vi "find_speedup.vi"(7 "Parameters":T2={"Stimulus"={"Type"=enum."Off", "Phase"=0.0, "Amplitude"=[], "Injection point"=enum."Total pose", "Closed loop"=FALSE, "Offset"=[], "Tip -> world"=FALSE, "Frequency"=0.0, "Length"=0.0}, "Goal Filter A"={"Speedup max"=0.0, "Speedup thresh"=0.0, "Speedup nonlin"=0.0, "Filters"=[]}, "Mode controls"={"Hold"=FALSE, "Cancellation"=FALSE, "Goal filter"=FALSE, "Trigger"=FALSE}, "Manipulator type"=enum."Current piezo", "Manipulator calibration"={"Tool offsets"=[[0.0, 0.0, 36200.0]], "Handle light calibration"=[], "Base pivots"=[], "Output pivots"=[], "Length center"=0.0, "Workspace height"=[], "Workspace diameter"=[0.0, 0.0, 36200.0], "Stack travel"=400.0, "Saturation pos"=375.0, "Inverse filters"=[], "Strut length"=0.0}, "Network"={"Remote Host"="", "Send Status"=FALSE, "Send Port"=0, "Recv Commands"=FALSE, "Recv Port"=0}, "Goal Filter B"={"Speedup max"=0.0, "Speedup thresh"=0.0, "Speedup nonlin"=0.0, "Filters"=[]}, "Cancellation"={"KP"={"XY"=0.0, "Rxy"=0.0, "Z"=0.0, "Rz"=0.0}, "KI"=0.0, "KD"={"XY"=0.0, "Rxy"=0.0, "Z"=0.0, "Rz"=0.0}, "Max vel"=20.0, "Max acc"=0.001, "Int error limit"=3.0, "RCM gain"=0.0, "Bypass"=FALSE, "Degraded gain"=0.0}, "Transition time"=0.0, "Estimation"={"Link"={"Measure noise"=[], "Process noise"=[], "Alt process noise"=[], "Alt turnoff cycles"=20, "Innovation limit"=[], "Residue threshold"=0.0, "Enable"=FALSE}, "Handle"={"Measure noise"=[], "Process noise"=[], "State limits"=[], "Innovation limit"=[], "Prediction Lookahead"=0.0, "Enable"=FALSE}}} {"Transition time" format="%_3f"; "Cancellation"."Degraded gain" min=0 max=1 step=0.1 format="%#_3p"; "Cancellation"."RCM gain" min=0 max=1 step=0.1 format="%#_3p"; "Cancellation"."KD"."Rz" min=-1 max=1 step=0.01 format="%#_3p"; "Cancellation"."KD"."Rxy" min=-1 max=1 step=0.01 format="%#_3p"; "Cancellation"."KD"."Z" min=-1 max=1 step=0.01 format="%#_3p"; "Cancellation"."KD"."XY" min=-1 max=1 step=0.01 format="%#_3p"; "Cancellation"."KI" min=0 max=1 step=0.01 format="%#_3p"; "Cancellation"."KP"."Rz" min=-1 max=1 step=0.01 format="%#_3p"; "Cancellation"."KP"."Rxy" min=-1 max=1 step=0.01 format="%#_3p"; "Cancellation"."KP"."Z" min=-1 max=1 step=0.01 format="%#_3p"; "Cancellation"."KP"."XY" min=-1 max=1 step=0.01 format="%#_3p"; "Cancellation"."Max acc" format="%#_3p"; "Goal Filter B"."Filters"."V limit range" format="%_3p"; "Goal Filter B"."Filters"."V limit" format="%_3p"; "Goal Filter B"."Filters"."Upper Q" format="%_3f"; "Goal Filter B"."Filters"."Upper Fc" format="%_3p"; "Goal Filter B"."Filters"."Lower Q" format="%_3f"; "Goal Filter B"."Filters"."Scale factor" format="%_3f"; "Goal Filter B"."Filters"."Lower Fc" format="%_3p"; "Goal Filter B"."Speedup nonlin" format="%_3p"; "Goal Filter B"."Speedup thresh" format="%_3p"; "Goal Filter B"."Speedup max" format="%_3p"; "Manipulator calibration"."Strut length" format="%#_4p"; "Manipulator calibration"."Saturation pos" format="%#.1f"; "Manipulator calibration"."Stack travel" format="%#.1f"; "Manipulator calibration"."Length center" format="%#_4p"; "Manipulator calibration"."Output pivots" format="%#_6f"; "Manipulator calibration"."Base pivots" format="%#_6f"; "Manipulator calibration"."Handle light calibration" format="%#.1f"; "Goal Filter A"."Filters"."V limit range" format="%_3p"; "Goal Filter A"."Filters"."V limit" format="%_3p"; "Goal Filter A"."Filters"."Upper Q" format="%_3f"; "Goal Filter A"."Filters"."Upper Fc" format="%_3p"; "Goal Filter A"."Filters"."Lower Q" format="%_3f"; "Goal Filter A"."Filters"."Scale factor" format="%_3f"; "Goal Filter A"."Filters"."Lower Fc" format="%_3p"; "Goal Filter A"."Speedup nonlin" format="%_3p"; "Goal Filter A"."Speedup thresh" format="%_3p"; "Goal Filter A"."Speedup max" format="%_3p"; "Stimulus"."Length" min=0.0 max=100.0 step=100.0 format="%#_4p"; "Stimulus"."Frequency" min=0.0 step=100.0 format="%#_4g"; "Stimulus"."Offset" format="%#_3p"; "Stimulus"."Amplitude" format="%#_3p"; "Stimulus"."Phase" min=-180.0 max=360.0 step=100.0 format="%#.2f"}, 9 "Goal Filter":T1={"Speedup max"=0.08, "Speedup thresh"=0.606, "Speedup nonlin"=3.0, "Filters"=[]} {"Filters"."V limit range" format="%_3p"; "Filters"."V limit" format="%_3p"; "Filters"."Upper Q" format="%_3f"; "Filters"."Upper Fc" format="%_3p"; "Filters"."Lower Q" format="%_3f"; "Filters"."Scale factor" format="%_3f"; "Filters"."Lower Fc" format="%_3p"; "Speedup nonlin" format="%_3p"; "Speedup thresh" format="%_3p"; "Speedup max" format="%_3p"}, 10 "Stack positions":sgl[](array[numeric])) -> (2 "Speedup":sgl)   [LabVIEW 2014]
uses:
  testing/Micron params.ctl
  testing/stimulus.ctl
  testing/injection_point.ctl
  goal_loop_parms.ctl
  testing/mode_conrols.ctl
  testing/manipulator_cal.ctl
  asap/labview/testing/probe_calibration.ctl
  host/network_params.ctl
  cancellation/sq_control_params.ctl
  cancellation/decoupled_gain.ctl
  cancellation/estimation_controls.ctl
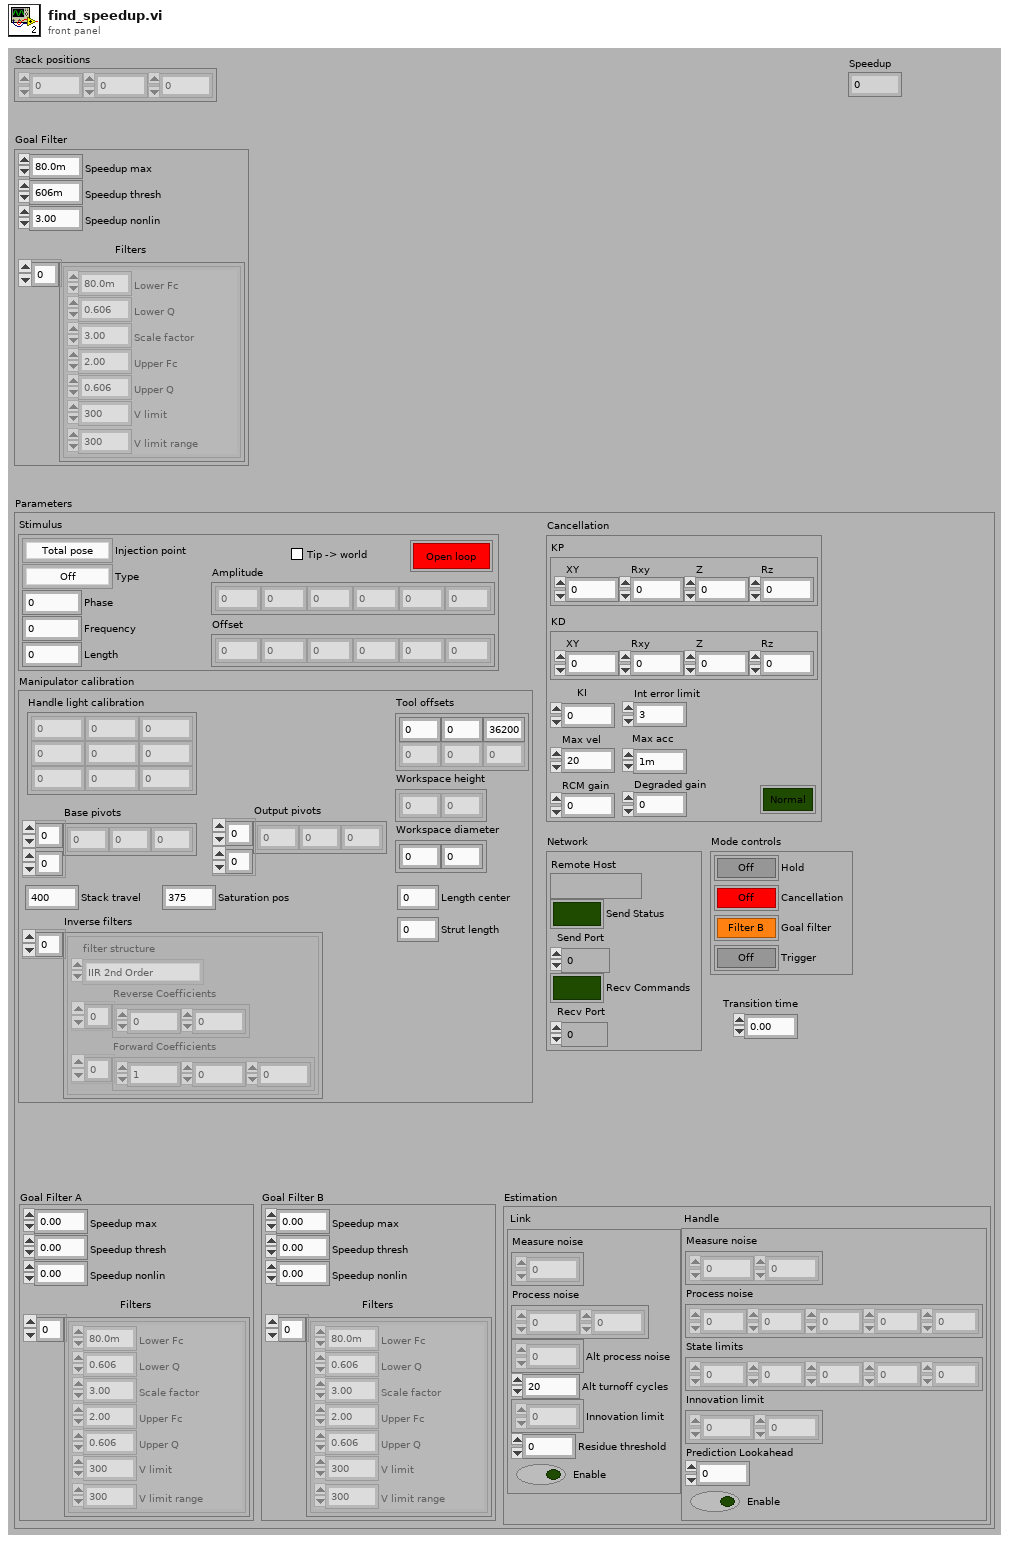
[diagram p1: front panel]
types:
  T1 = typedef "goal_loop_parms.ctl" = cluster{"Speedup max":sgl, "Speedup thresh":sgl, "Speedup nonlin":sgl, "Filters":cluster{"Lower Fc":sgl, "Lower Q":sgl, "Scale factor":sgl, "Upper Fc":sgl, "Upper Q":sgl, "V limit":sgl, "V limit range":sgl}[]}
  T2 = typedef "Micron params.ctl" = cluster{"Stimulus":T3, "Goal Filter A":T1, "Mode controls":T5, "Manipulator type":enum16{"Current piezo", "Voltage piezo"}, "Manipulator calibration":T6, "Network":T8, "Goal Filter B":T1, "Cancellation":T9, "Transition time":sgl, "Estimation":T11}
  T3 = typedef "stimulus.ctl" = cluster{"Type":enum16{"Off", "Step", "Sine", "Triangle", "Arbitrary"}, "Phase":dbl, "Amplitude":sgl[], "Injection point":T4, "Closed loop":bool, "Offset":sgl[], "Tip -> world":bool, "Frequency":dbl, "Length":dbl}
  T4 = typedef "injection_point.ctl" = enum16{"Total pose", "V limiter", "Goal ", "Link position", "KF link position", "Inverse kin", "Link goal", "Link error", "Controller", "Output", "Drive", "Light"}
  T5 = typedef "mode_conrols.ctl" = cluster{"Hold":bool, "Cancellation":bool, "Goal filter":bool, "Trigger":bool}
  T6 = typedef "manipulator_cal.ctl" = cluster{"Tool offsets":sgl[][], "Handle light calibration":T7, "Base pivots":sgl[][], "Output pivots":sgl[][], "Length center":sgl, "Workspace height":sgl[], "Workspace diameter":sgl[], "Stack travel":sgl, "Saturation pos":sgl, "Inverse filters":cluster{"filter structure":enum32{"IIR 2nd Order", "IIR 4th Order"}, "Reverse Coefficients":dbl[], "Forward Coefficients":dbl[]}[], "Strut length":sgl}
  T7 = typedef "probe_calibration.ctl" = sgl[][]
  T8 = typedef "network_params.ctl" = cluster{"Remote Host":string, "Send Status":bool, "Send Port":u16, "Recv Commands":bool, "Recv Port":u16}
  T9 = typedef "sq_control_params.ctl" = cluster{"KP":T10, "KI":sgl, "KD":T10, "Max vel":sgl, "Max acc":sgl, "Int error limit":sgl, "RCM gain":sgl, "Bypass":bool, "Degraded gain":sgl}
  T10 = typedef "decoupled_gain.ctl" = cluster{"XY":sgl, "Rxy":sgl, "Z":sgl, "Rz":sgl}
  T11 = typedef "estimation_controls.ctl" = cluster{"Link":cluster{"Measure noise":dbl[], "Process noise":dbl[], "Alt process noise":dbl[], "Alt turnoff cycles":i32, "Innovation limit":dbl[], "Residue threshold":dbl, "Enable":bool}, "Handle":cluster{"Measure noise":dbl[], "Process noise":dbl[], "State limits":dbl[], "Innovation limit":dbl[], "Prediction Lookahead":sgl, "Enable":bool}}
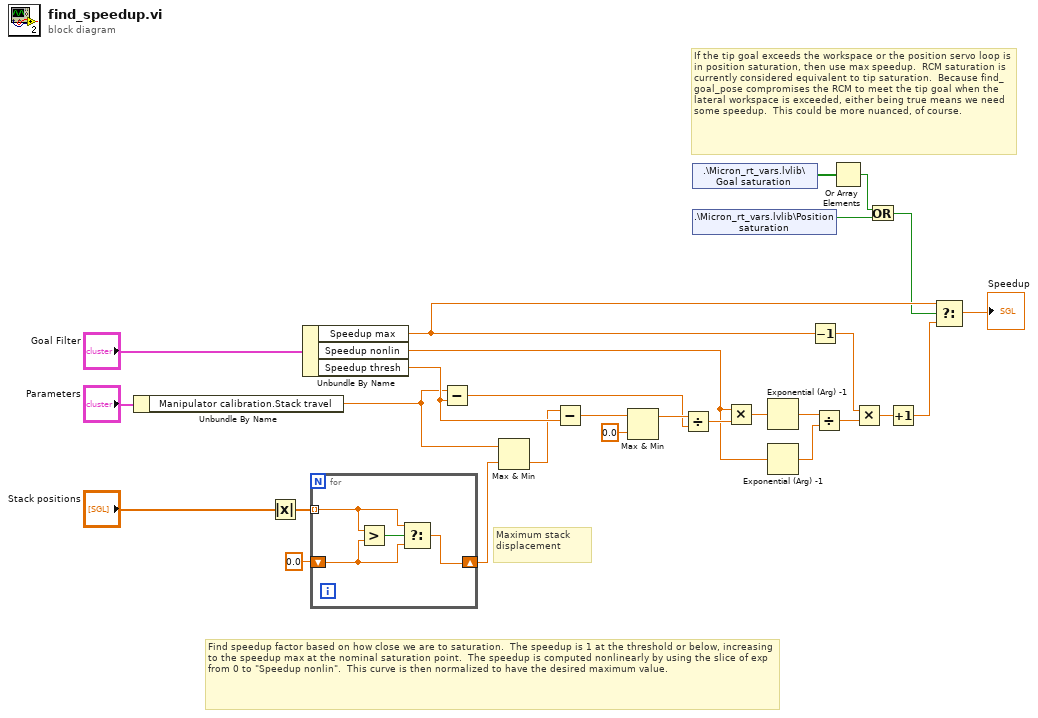
[diagram p0: block diagram]
diagram:
  # "If the tip goal exceeds the workspace or the position servo loop is in position saturation, then use max speedup.  RCM saturation is currently considered equivalent to tip saturation.  Because find_goal_pose compromises the RCM to meet the tip goal when the lateral workspace is exceeded, either being true means we need some speedup.  This could be more nuanced, of course."
  # "Find speedup factor based on how close we are to saturation.  The speedup is 1 at the threshold or below, increasing to the speedup max at the nominal saturation point.  The speedup is computed nonlinearly by using the slice of exp from 0 to \"Speedup nonlin\".  This curve is then normalized to have the desired maximum value."
  # "Maximum stack displacement"
  n1 = Unbundle By Name("Parameters") -> ("Manipulator calibration.Stack travel"=w5:sgl)
  n2 = Absolute Value(x="Stack positions") -> (abs(x)=w27:sgl[])
  n3 = Unbundle By Name("Goal Filter") -> ("Speedup max"=w10:sgl, "Speedup nonlin"=w18:sgl, "Speedup thresh"=w23:sgl)
  n4 = for {
    tunnel: w27 -> [w31] mode=indexing
    shift-right: [w29] -> w9
    shift-left: sgl 0.0 ("Goal Filter.Speedup thresh") -> [w30]
    n5 = Greater?(x=w31, y=w30) -> (0:w32:bool)
    n6 = Select(t=w31, s=w32, f=w30) -> (s? t:f=w29:sgl)
  }
  n7 = Subtract(x=w5, y=w23) -> (x-y=w14:sgl)
  n8 = Max & Min(x=w5, y=w9) -> (min(x,y)=w8:sgl)  [unwired: 1 out]
  n9 = Subtract(x=w8, y=w23) -> (x-y=w22:sgl)
  n10 = Max & Min(x=w22, y=sgl 0.0) -> (max(x,y)=w21:sgl)  [unwired: 1 out]
  n11 = Divide(x=w21, y=w14) -> (x/y=w20:sgl)
  n12 = shared-variable ".\\Micron_rt_vars.lvlib\\Goal saturation"() -> (w2:bool[])  [unwired: 2 out]
  n13 = shared-variable ".\\Micron_rt_vars.lvlib\\Position saturation"() -> (w4:bool)  [unwired: 2 out]
  n14 = Multiply(x=w18, y=w20) -> (x*y=w19:sgl)
  n15 = Exponential (Arg) -1(1:w19) -> (0:w17:sgl)
  n16 = Exponential (Arg) -1(1:w18) -> (0:w16:sgl)
  n17 = Decrement(x=w10) -> (x-1=w11:sgl)
  n18 = Divide(x=w17, y=w16) -> (x/y=w15:sgl)
  n19 = Or Array Elements(Boolean array=w2) -> (logical OR=w1:bool)
  n20 = Multiply(x=w11, y=w15) -> (x*y=w13:sgl)
  n21 = Or(x=w1, y=w4) -> (x .or. y?=w3:bool)
  n22 = Increment(x=w13) -> (x+1=w12:sgl)
  n23 = Select(t=w10, s=w3, f=w12) -> (s? t:f=→"Speedup":sgl)
